vi "Lockin.DAQ.Start.AI.vi"(6 "error in (no error)":errorcluster, 9 "Lockin.DAQ in":refnum<class "Instrument.DAQ.lvclass">) -> (0 "error out":errorcluster, 3 "Lockin.DAQ out":refnum<class "Instrument.DAQ.lvclass">)   [LabVIEW 2019, in "Instrument.DAQ.lvclass"]
uses:
  Instrument.DAQ.lvclass
  Instrument.DAQ.lvclass/Instrument.DAQ.ctl
  <vilib>/DAQmx/read.llb/DAQmx Read (Analog 1D Wfm NChan NSamp).vi
  <vilib>/DAQmx/miscellaneous.llb/DAQmx Fill In Error Info.vi
  <resource>/objmgr/daqmx.rc
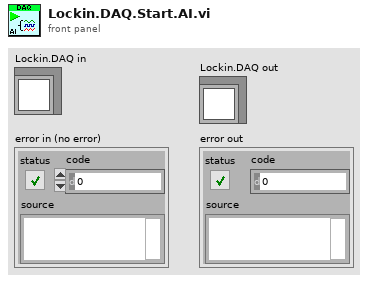
[diagram p1: front panel]
types:
  T1 = typedef "Instrument.DAQ.lvclass/DAQ.Type--enum.ctl" = enum16{"None", "USB 4431", "PXI 446x"}
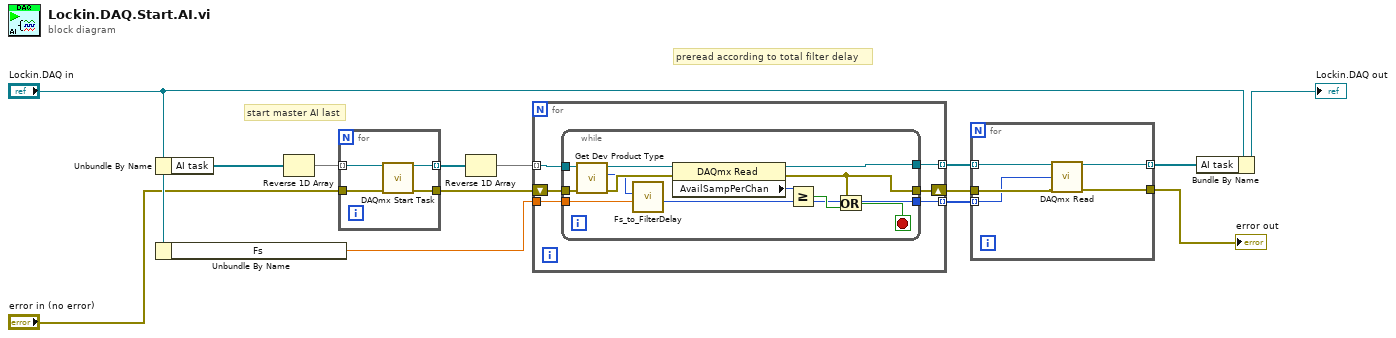
[diagram p0: block diagram]
diagram:
  # "preread according to total filter delay"
  # "start master AI last"
  n1 = Unbundle By Name("Lockin.DAQ in") -> ("AI task"=w12:refnum<k21>[])
  n2 = Unbundle By Name("Lockin.DAQ in") -> ("Fs"=w8:dbl)
  n3 = Reverse 1D Array(array=w12) -> (reversed array=w11:refnum<k21>[])
  n4 = for {
    tunnel: w11 -> [w18] mode=indexing
    tunnel: "error in (no error)" -> [w17]
    tunnel: [w16] -> w10 mode=indexing
    tunnel: [w15] -> w9
    n5 = call <vilib>:"DAQmx Start Task.vi"("task/channels in"=w18, "error in"=w17) -> ("task out"=w16:refnum<k21>, "error out"=w15:errorcluster)  [unwired: 12 in]
  }
  n6 = Reverse 1D Array(array=w10) -> (reversed array=w1:refnum<k21>[])
  n7 = for {
    tunnel: w1 -> [w24] mode=indexing
    tunnel: w8 -> [w22]
    shift-right: [w21] -> w5
    shift-left: w9 -> [w23]
    tunnel: [w20] -> w7 mode=indexing
    tunnel: [w19] -> w6 mode=indexing
    n8 = while {
      tunnel: w24 -> [w36]
      tunnel: w23 -> [w35]
      tunnel: w22 -> [w34]
      tunnel: [w28] -> w21
      tunnel: [w27] -> w20
      tunnel: [w26] -> w19
      stop <- w30 stop-if-true
      n9 = call "Get Dev Product Type.vi"("error in (no error)"=w35, "Refnum in"=w36) -> ("error out"=w29:errorcluster, "DAQ Type"=w25:T1, "Refnum out"=w33:refnum<k21>)  [unwired: 6 in, 1 out]
      n10 = call "Fs_to_FilterDelay.vi"("Fs"=w34, "DAQ Type"=w25) -> ("Total Filter Delay (samples)"=w27:i32)  [unwired: 9 in]
      n11 = property class="DAQmx Read"(reference=w33, error in=w29) -> (reference out=w26:refnum<k21>, error out=w28:errorcluster, "AvailSampPerChan"=w32:u32)
      n12 = Greater Or Equal?(x=w32, y=w27) -> (x >= y?=w31:bool)
      n13 = Or(x=w28, y=w31) -> (x .or. y?=w30:bool)
    }
  }
  n14 = for {
    tunnel: w7 -> [w39] mode=indexing
    tunnel: w6 -> [w41] mode=indexing
    tunnel: w5 -> [w40]
    tunnel: [w38] -> w3
    tunnel: [w37] -> w4 mode=indexing
    n15 = call-poly <vilib>:"DAQmx Read.vi"("task/channels in"=w41, "number of samples per channel"=w39, "error in"=w40) -> ("task out"=w37:refnum<k21>, "error out"=w38:errorcluster)  [unwired: 10 in, 1 out]
  }
  "error out" <- w3
  n16 = Bundle By Name(cluster="Lockin.DAQ in", "AI task"=w4) -> (→"Lockin.DAQ out":refnum<class "Instrument.DAQ.lvclass">)
